vi "Memory.Array.Numeric.Count to Size.vi"(8 "error in (no error)":errorcluster, 10 "count":u64, 11 "Numeric Array in":refnum<class "Memory.Array.Numeric.lvclass">) -> (0 "error out":errorcluster, 2 "size":u64 format="%d bytes", 3 "Numeric Array out":refnum<class "Memory.Array.Numeric.lvclass">)   [LabVIEW 2016, in "LabVIEW Memory Manager.lvlib" / "Memory.Array.Numeric.lvclass"]
uses:
  Memory.Array.Numeric.lvclass
  Memory.Array.Numeric.lvclass/Memory.Array.Numeric.ctl
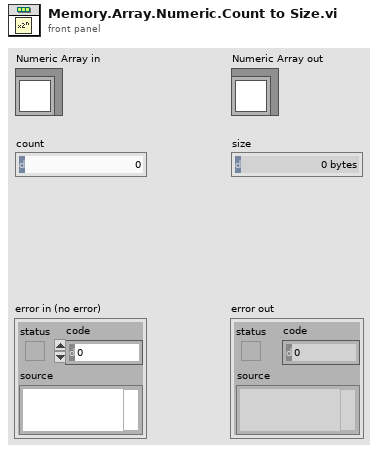
[diagram p1: front panel]
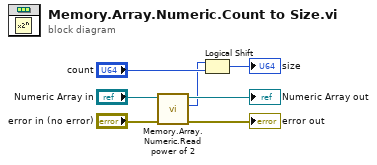
[diagram p0: block diagram]
diagram:
  n1 = call "Memory.Array.Numeric.Read power of 2.vi"("error in (no error)"="error in (no error)", "Numeric Array in"="Numeric Array in") -> ("error out"=→"error out":errorcluster, "power of 2"=w1:i16, "Numeric Array out"=→"Numeric Array out":refnum<class "Memory.Array.Numeric.lvclass">)  [unwired: 7 in]
  n2 = Logical Shift(y=w1, x="count") -> (x << y=→"size":u64)
